vi "revise data years.vi"(11 "Array in":string[][](array[string])) -> (3 "Array out":string[][](array[string]))   [LabVIEW 2018]
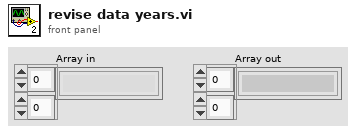
[diagram p1: front panel]
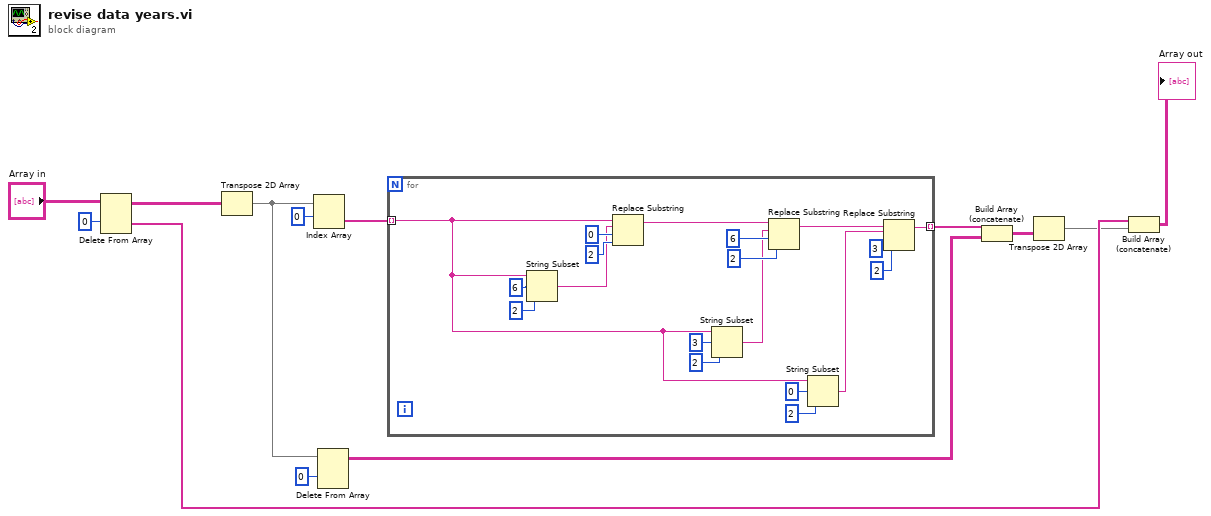
[diagram p0: block diagram]
diagram:
  n1 = Delete From Array(array="Array in", index (row)=0) -> (deleted portion=w12:string[], array with subset deleted=w9:string[][])  [unwired: 2 in]
  n2 = Transpose 2D Array(2D array=w9) -> (transposed array=w4:string[][])
  n3 = Index Array(array=w4, index (row)=0) -> (element=w2:string[])  [unwired: 1 in]
  n4 = Delete From Array(array=w4, index (row)=0) -> (array with subset deleted=w6:string[][])  [unwired: 2 in, 1 out]
  n5 = for {
    tunnel: w2 -> [w14] mode=indexing
    tunnel: [w16] -> w3 mode=indexing
    n6 = String Subset(string=w14, offset (0)=6, length (rest)=2 ("length (rest)")) -> (substring=w28:string)
    n7 = Replace Substring(2:2 ("length (len. of substring)"), 3:0 ("offset (0)"), 4:w28, 5:w14) -> (1:w27:string)  [unwired: 1 out]
    n8 = String Subset(string=w14, offset (0)=3, length (rest)=2 ("length (rest)")) -> (substring=w22:string)
    n9 = Replace Substring(2:2 ("length (len. of substring)"), 3:6 ("offset (0)"), 4:w22, 5:w27) -> (1:w21:string)  [unwired: 1 out]
    n10 = String Subset(string=w14, offset (0)=0, length (rest)=2 ("length (rest)")) -> (substring=w15:string)
    n11 = Replace Substring(2:2 ("length (len. of substring)"), 3:3 ("offset (0)"), 4:w15, 5:w21) -> (1:w16:string)  [unwired: 1 out]
  }
  n12 = Build Array (concatenate)(w3, w6) -> (w7:string[][])
  n13 = Transpose 2D Array(2D array=w7) -> (transposed array=w10:string[][])
  n14 = Build Array (concatenate)(w12, w10) -> (→"Array out":string[][])
